vi "Decoder.vi"(8 "error in (no error)":errorcluster, 11 "ISO 14443 A DOWN in":refnum<class "ISO 14443 A DOWN.lvclass">) -> (0 "error out":errorcluster, 3 "ISO 14443 A DOWN out":refnum<class "ISO 14443 A DOWN.lvclass">)   [LabVIEW 2019, in "ISO 14443 A DOWN.lvclass"]
uses:
  ISO 14443 A DOWN.lvclass
  TypeDef/Store.ctl
  ISO 14443 A DOWN.lvclass/ISO 14443 A DOWN.ctl
  RFID system.lvclass
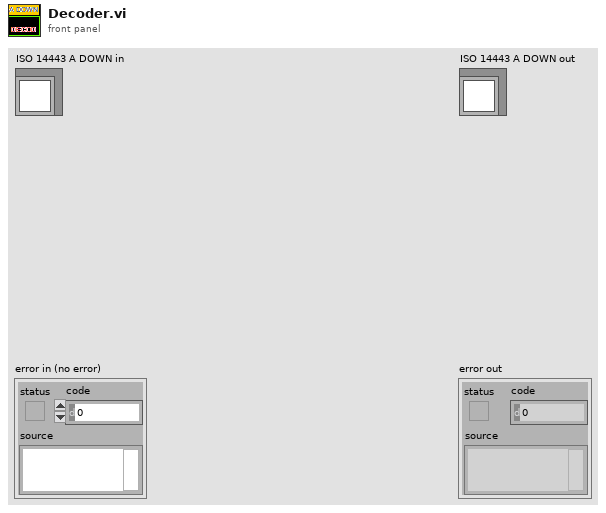
[diagram p1: front panel]
types:
  T1 = typedef "Store.ctl" = enum16{"envelope", "noise", "demSubCar", "CH_frame", "Decode", "demodulate", "in", "out", "sum", "subCarrier", "frame", "command", "encode", "modulate", "encode_UP", "modulate_up", "demod_up", "envelop_up", "sum_up", "out_up", "in_up"}
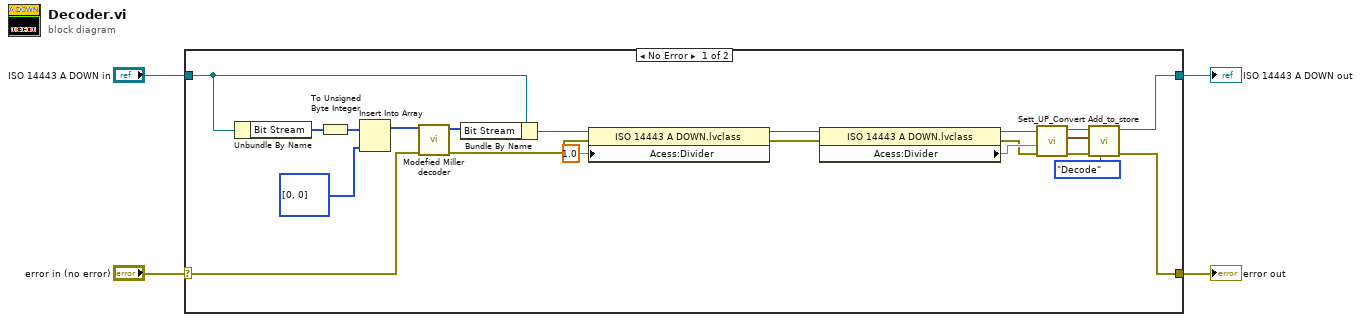
[diagram p0: block diagram]
diagram:
  n1 = case shown="No Error" "error in (no error)" {
    selector: "error in (no error)" -> [w21 w27]
    tunnel: [w15 w27] -> w3
    tunnel: "ISO 14443 A DOWN in" -> [w19 w26]
    tunnel: [w16 w26] -> w1
    frame No Error {
      n2 = Unbundle By Name(w19) -> ("Bit Stream"=w22:u8[])
      n3 = To Unsigned Byte Integer(number=w22) -> (unsigned 8bit integer=w25:u8[])
      n4 = Insert Into Array(array=w25, new element=u8[] [0, 0]) -> (w24:u8[])  [unwired: 1 in]
      n5 = call "Modefied Miller decoder.vi"("error in (no error)"=w21, "Bit stream in"=w24) -> ("error out"=w7:errorcluster, "output array"=w20:u8[])  [unwired: 8 in]
      n6 = Bundle By Name(cluster=w19, "Bit Stream"=w20) -> (w18:refnum<class "ISO 14443 A DOWN.lvclass">)
      n7 = property class="ISO 14443 A DOWN.lvclass"(reference=w18, error in=w7, "Acess:Divider"=1.0 ("Divider")) -> (reference out=w8:refnum<class "ISO 14443 A DOWN.lvclass">, error out=w6:errorcluster)
      n8 = property class="ISO 14443 A DOWN.lvclass"(reference=w8, error in=w6) -> (reference out=w11:refnum<class "ISO 14443 A DOWN.lvclass">, error out=w9:errorcluster, "Acess:Divider"=w10:dbl)
      n9 = call-dynamic "Sett_UP_Convert.vi"("error in (no error)"=w9, "Divider(1)"=w10, "ISO 14443 A DOWN in"=w11) -> ("error out"=w14:errorcluster, "Waveform"=w13:waveform(dbl), "ISO 14443 A DOWN out"=w17:refnum<class "ISO 14443 A DOWN.lvclass">)  [unwired: 6 in]
      n10 = call "Add_to_store.vi"("Store"=Store."Decode", "error in (no error)"=w14, "Waveform"=w13, "RFID system in"=w17) -> ("error out"=w15:errorcluster, "RFID system out"=w16:refnum<class "ISO 14443 A DOWN.lvclass">)  [unwired: 6 in]
    }
    frame Error {
    }
  }
  "error out" <- w3
  "ISO 14443 A DOWN out" <- w1
